vi "Duty Cycle Absolute Encoder.vi"() -> ()   [LabVIEW 2025]
doc: "This example shows how to configure and read values from an absolute encoder that has PWM duty cycle output.\n\nIt will display the raw encoder value, absolute angle, cumulative angle, and revolutions.\n\nThis example expects a USB cable connected from your development PC to the Type B USB Jack (next to the power input) on the roboRIO."
uses:
  <vilib>/Rock Robotics/SystemInterfaces/DIO/FPGA_DIOChannel.ctl
  <vilib>/Rock Robotics/SystemInterfaces/AnalogTrigger/FPGA_AnalogTriggerOutType.ctl
  <vilib>/Rock Robotics/WPI/Counter/WPI_CounterDigitalInputToDigitalSource.vi
  <vilib>/Rock Robotics/WPI/AnalogTrigger/WPI_AnalogTriggerOpen_DutyCycle.vi
  <vilib>/Rock Robotics/WPI/Counter/WPI_CounterAnalogTriggerToDigitalSource.vi
  <vilib>/Rock Robotics/WPI/Counter/WPI_CounterOpen UpDown Mode.vi
panel:
  out "Cumulative Angle":dbl
  out "Absolute Angle":dbl(knob) scale=0.0..360.0
  out "Revolutions":i32
  out "Raw Output":dbl
  in  "Channel":T1
  in  "stop":bool
  # "Set this input before running."
  # "Output information."
  # "Absolute Encoder\nDuty Cycle (PWM)"
  # "This shows wiring for a generic absolute encoder with duty cycle PWM output.  Some encoders may have G labeled as Com.  Some may have +5V labeled as +VDC."
  # "Encoder\nG (brown wire)--------\n+5V (orange wire)-----\nPWM (blue wire)------"
  # "roboRIO\nDIO-0 \nDIO-0  5V\nDIO-0  S"
  # "PWM"
  # "+5V"
  # "G"
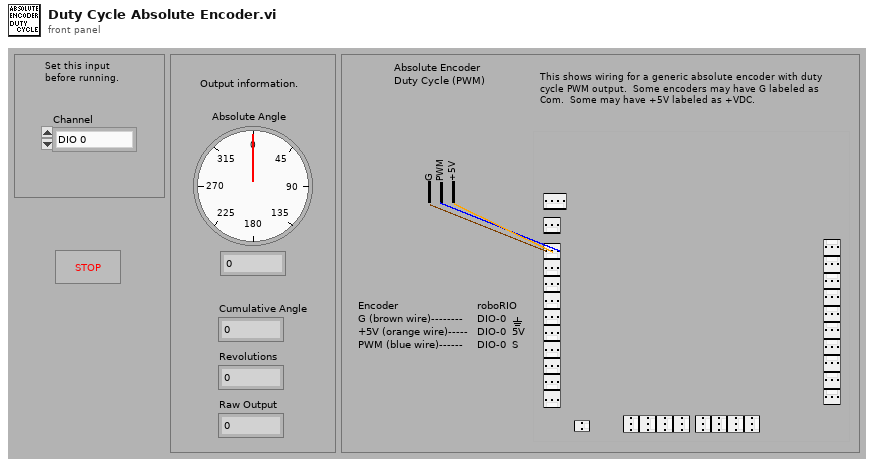
[diagram p1: front panel]
types:
  T1 = typedef "FPGA_DIOChannel.ctl" = enum8{"DIO 0", "DIO 1", "DIO 2", "DIO 3", "DIO 4", "DIO 5", "DIO 6", "DIO 7", "DIO 8", "DIO 9", "DIO MXP 0", "DIO MXP 1", "DIO MXP 2", "DIO MXP 3", "DIO MXP 4", "DIO MXP 5", "DIO MXP 6", "DIO MXP 7", "DIO MXP 8", "DIO MXP 9", "DIO MXP 10", "DIO MXP 11", "DIO MXP 12", "DIO MXP 13", "DIO MXP 14", "DIO MXP 15", "SPI Port CS1", "SPI Port CS2", "SPI Port CS3", "SPI Port MISO", "SPI Port MOSI", "Invalid"}
  T2 = enum16{"Rising Edge", "Falling Edge", "Raising & Falling Edge", "Disabled"}
  T3 = typedef "FPGA_AnalogTriggerOutType.ctl" = enum16{"InWindow", "TriggerState", "Rising", "Falling"}
  T4 = typedef "WPI_DigitalInputDevRef.ctl" = cluster{"DevStatus":errorcluster, "DIO Channel":T1}
  T5 = typedef "FPGA_CounterEncoderSourceConvertionLVSourceType.ctl" = cluster{"DevStatus":errorcluster, "AnalogTriggerMode?":bool, "DigitalMode":cluster{"DIO Channel":T6}, "AnalogTriggerMode":cluster{"AnalogTriggerIndex":T7, "OutputType":T3}}
  T6 = typedef "FPGA_DIODigitalSourceChannel.ctl" = enum8{"DIO 0", "DIO 1", "DIO 2", "DIO 3", "DIO 4", "DIO 5", "DIO 6", "DIO 7", "DIO 8", "DIO 9", "DIO MXP 0", "DIO MXP 1", "DIO MXP 2", "DIO MXP 3", "DIO MXP 4", "DIO MXP 5", "DIO MXP 6", "DIO MXP 7", "DIO MXP 8", "DIO MXP 9", "DIO MXP 10", "DIO MXP 11", "DIO MXP 12", "DIO MXP 13", "DIO MXP 14", "DIO MXP 15", "SPI Port CS1", "SPI Port CS2", "SPI Port CS3", "SPI Port MISO", "SPI Port MOSI", "Disabled"}
  T7 = typedef "FPGA_AnalogTriggerIndex.ctl" = enum8{"Trig 0", "Trig 1", "Trig 2", "Trig 3", "Trig 4", "Trig 5", "Trig 6", "Trig 7", "Invalid"}
  T8 = typedef "FPGA_DutyCycleDevRef.ctl" = cluster{"DevStatus":errorcluster, "DutyCycleIndex":T9}
  T9 = typedef "FPGA_DutyCycleIndex.ctl" = enum8{"DutyCycle 0", "DutyCycle 1", "DutyCycle 2", "DutyCycle 3", "DutyCycle 4", "DutyCycle 5", "DutyCycle 6", "DutyCycle 7", "Invalid"}
  T10 = typedef "FPGA_AnalogTriggerDevRef.ctl" = cluster{"DevStatus":errorcluster, "AnalogTriggerIndex":T7}
  T11 = typedef "WPI_CounterDevRef.ctl" = cluster{"DevStatus":errorcluster, "CntIndex":T12}
  T12 = typedef "FPGA_CounterCtrSystemIndex.ctl" = enum8{"Ctr 0", "Ctr 1", "Ctr 2", "Ctr 3", "Ctr 4", "Ctr 5", "Ctr 6", "Ctr 7", "Invalid"}
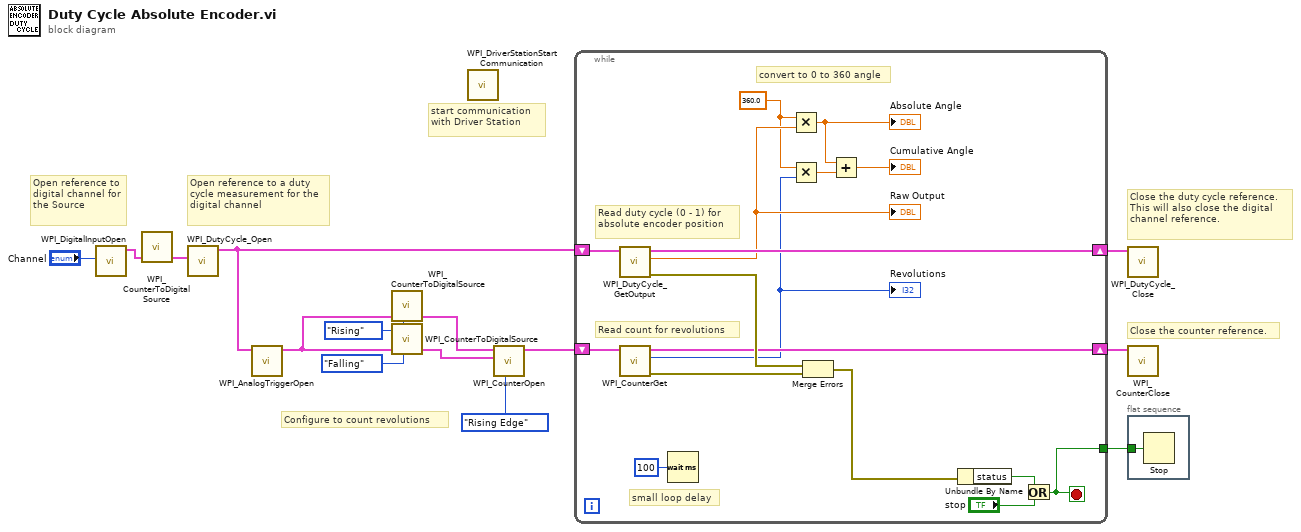
[diagram p0: block diagram]
diagram:
  # "Close the counter reference."
  # "Configure to count revolutions"
  # "start communication with Driver Station"
  # "Close the duty cycle reference.\nThis will also close the digital \nchannel reference."
  # "Open reference to a duty cycle measurement for the digital channel"
  # "Open reference to digital channel for the Source"
  n1 = call <vilib>:"WPI_DigitalInputOpen.vi"("DIO Channel"="Channel") -> ("DigitalInputDevRef"=w13:T4)  [unwired: 1 in, 9 out]
  n2 = call-poly <vilib>:"WPI_CounterToDigitalSource.vi"("DigitalInputDevRef"=w13) -> ("Digital Source"=w14:T5)  [unwired: 6 out]
  n3 = call <vilib>:"WPI_DutyCycle_Open.vi"("Source"=w14) -> ("DutyCycleDevRef"=w5:T8)  [unwired: 9 in, 1 out]
  n4 = call-poly <vilib>:"WPI_AnalogTriggerOpen.vi"("AnalogTriggerSource"=w5) -> ("AnalogTriggerDevRef"=w6:T10)  [unwired: 9 in, 1 out]
  n5 = call-poly <vilib>:"WPI_CounterToDigitalSource.vi"("AnalogTriggerDevRef"=w6, "OutputType"=FPGA_AnalogTriggerOutType."Rising") -> ("Digital Source"=w10:T5)  [unwired: 5 out]
  n6 = call-poly <vilib>:"WPI_CounterToDigitalSource.vi"("AnalogTriggerDevRef"=w6, "OutputType"=FPGA_AnalogTriggerOutType."Falling") -> ("Digital Source"=w7:T5)  [unwired: 5 out]
  n7 = call <vilib>:"WPI_DriverStationStart Communication.vi"() -> ()  [unwired: 3 in, 9 out]
  n8 = call-poly <vilib>:"WPI_CounterOpen.vi"("DownEdge"=T2."Rising Edge", "Down Source"=w7, "Up Source"=w10) -> ("CounterDevRef"=w4:T11)  [unwired: 4 in, 4 out]
  n9 = while {
    shift-right: [w25] -> w3
    shift-left: w5 -> [w27]
    tunnel: [w30] -> w11
    shift-right: [w21] -> w2
    shift-left: w4 -> [w26]
    stop <- w30 stop-if-true
    w19 = 360.0 ("x")
    # "Read count for revolutions"
    # "Read duty cycle (0 - 1) for absolute encoder position"
    # "convert to 0 to 360 angle"
    # "small loop delay"
    n10 = call <vilib>:"WPI_DutyCycle_GetOutput.vi"("DutyCycleDevRef"=w27) -> ("error out"=w23:errorcluster, "Output"=w20:dbl, "DutyCycleDevRef Out"=w25:T8)  [unwired: 8 in]
    "Raw Output" <- w20
    n11 = call <vilib>:"WPI_CounterGet.vi"("CounterDevRef in"=w26) -> ("error out"=w24:errorcluster, "Value"=w18:i32, "CounterDevRef out"=w21:T11)  [unwired: 5 in, 3 out]
    "Revolutions" <- w18
    n12 = Wait (ms)(milliseconds to wait=u32 100) -> ()  [unwired: 1 out]
    n13 = Multiply(x=w19, y=w20) -> (x*y=w16:dbl)
    "Absolute Angle" <- w16
    n14 = Multiply(x=w19, y=w18) -> (x*y=w17:dbl)
    n15 = Merge Errors(w23, w24) -> (w22:errorcluster)
    n16 = Add(x=w16, y=w17) -> (x+y=→"Cumulative Angle":dbl)
    n17 = Unbundle By Name(w22) -> ("status"=w28:bool)
    n18 = Or(x=w28, y="stop") -> (x .or. y?=w30:bool)
  }
  n19 = call <vilib>:"WPI_DutyCycle_Close.vi"("DutyCycleDevRef"=w3) -> ()  [unwired: 10 in, 1 out]
  n20 = call <vilib>:"WPI_CounterClose.vi"("CounterDevRef"=w2) -> ()  [unwired: 10 in, 1 out]
  n21 = flat-sequence {
    tunnel: w11 -> [w32]
    frame #0 {
      n22 = Stop(stop? (T)=w32) -> ()
    }
  }
